vi "ParaChange.vi"(10 "新段名":string, 11 "原段名":string) -> ()   [LabVIEW 2020]
uses:
  <vilib>/Utility/config.llb/Read Key (String).vi
  <vilib>/Utility/config.llb/Write Key (String).vi
  <vilib>/Utility/config.llb/NI_LVConfig.lvlib
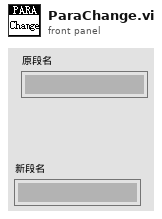
[diagram p1: front panel]
types:
  T1 = typedef "NI_LVConfig.lvlib/Config Data RefNum.ctl" = refnum<k1>
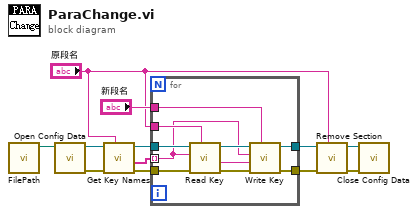
[diagram p0: block diagram]
diagram:
  n1 = call "FilePath.vi"() -> ("添加的路径"=w12:path)  [unwired: 11 in]
  n2 = call <vilib>:"Open Config Data.vi"("configuration file path"=w12) -> ("error out"=w10:errorcluster, "refnum"=w11:T1)  [unwired: 8 in, 1 out]
  n3 = call <vilib>:"Get Key Names.vi"("section"="原段名", "error in (no error)"=w10, "refnum"=w11) -> ("error out"=w7:errorcluster, "key names"=w8:string[], "refnum out"=w9:T1)  [unwired: 5 in, 1 out]
  n4 = for {
    tunnel: w9 -> [w19]
    tunnel: w8 -> [w14] mode=indexing
    tunnel: w7 -> [w18]
    tunnel: "新段名" -> [w22]
    tunnel: "原段名" -> [w21]
    tunnel: [w16] -> w5
    tunnel: [w15] -> w4
    n5 = call-poly <vilib>:"Read Key.vi"("section"=w21, "error in (no error)"=w18, "key"=w14, "refnum"=w19) -> ("error out"=w17:errorcluster, "value"=w13:string, "refnum out"=w20:T1)  [unwired: 4 in, 1 out]
    n6 = call-poly <vilib>:"Write Key.vi"("section"=w22, "error in (no error)"=w17, "value"=w13, "key"=w14, "refnum"=w20) -> ("error out"=w15:errorcluster, "refnum out"=w16:T1)  [unwired: 4 in, 1 out]
  }
  n7 = call <vilib>:"Remove Section.vi"("section"="原段名", "error in (no error)"=w4, "refnum"=w5) -> ("error out"=w1:errorcluster, "refnum out"=w2:T1)  [unwired: 6 in, 1 out]
  n8 = call <vilib>:"Close Config Data.vi"("error in (no error)"=w1, "refnum"=w2) -> ()  [unwired: 8 in, 2 out]
